vi "Menu Act Language.vi"(8 "error in (no error)":errorcluster, 10 "Language Name":string, 11 "LF2R IDE in":refnum<class "LF2R IDE.lvclass">) -> (0 "error out":errorcluster, 3 "LF2R IDE out":refnum<class "LF2R IDE.lvclass">)   [LabVIEW 2018, in "LF2R IDE.lvlib" / "LF2R IDE.lvclass"]
uses:
  LF2R IDE.lvclass
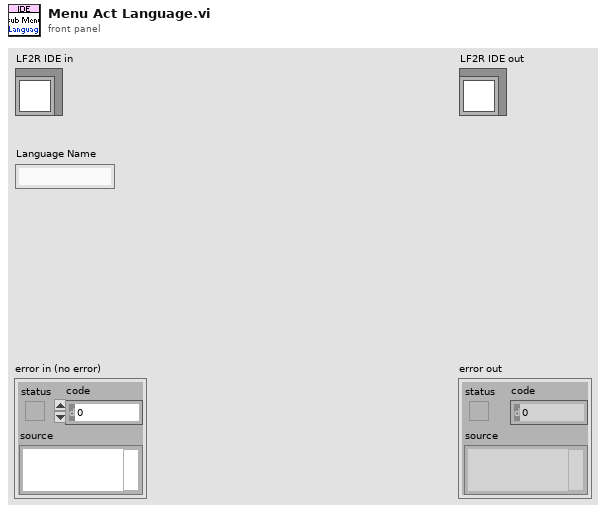
[diagram p1: front panel]
types:
  T1 = typedef "LF2R IDE.lvlib/LF2R IDE.lvclass/Const UI Description Setting.ctl" = cluster{"Title":T2, "Frame Basic":T4, "Frame Skill":T5, "bp":T6, "w":T7, "b":T8, "i":T9, "o":T10, "c":T11, "Other":T12}
  T2 = typedef "LF2R IDE.lvlib/LF2R IDE.lvclass/Const UI Desc Frame Title.ctl" = cluster{"Frame Num":T3, "Name":T3}
  T3 = typedef "LF2R IDE.lvlib/LF2R IDE.lvclass/Const UI Desc Property.ctl" = cluster{"Name":string, "Tip":string}
  T4 = typedef "LF2R IDE.lvlib/LF2R IDE.lvclass/Const UI Desc Frame Basic.ctl" = cluster{"pic":T3, "state":T3, "wait":T3, "next":T3, "dvx":T3, "dvy":T3, "dvz":T3, "centerx":T3, "centery":T3, "sound":T3}
  T5 = typedef "LF2R IDE.lvlib/LF2R IDE.lvclass/Const UI Desc Frame Skill.ctl" = cluster{"mp":T3, "hit_a":T3, "hit_d":T3, "hit_j":T3, "hit_Fa":T3, "hit_Ua":T3, "hit_Da":T3, "hit_Fj":T3, "hit_Uj":T3, "hit_Dj":T3, "hit_ja":T3}
  T6 = typedef "LF2R IDE.lvlib/LF2R IDE.lvclass/Const UI Desc Frame bp.ctl" = cluster{"x":T3, "y":T3}
  T7 = typedef "LF2R IDE.lvlib/LF2R IDE.lvclass/Const UI Desc Frame w.ctl" = cluster{"kind":T3, "x":T3, "y":T3, "weaponact":T3, "cover":T3, "dvx":T3, "dvy":T3, "dvz":T3, "attacking":T3}
  T8 = typedef "LF2R IDE.lvlib/LF2R IDE.lvclass/Const UI Desc Frame b.ctl" = cluster{"kind":T3, "x":T3, "y":T3, "w":T3, "h":T3, "index":T3}
  T9 = typedef "LF2R IDE.lvlib/LF2R IDE.lvclass/Const UI Desc Frame i.ctl" = cluster{"kind":T3, "x":T3, "y":T3, "w":T3, "h":T3, "zwidth":T3, "dvx":T3, "dvy":T3, "dvz":T3, "fall":T3, "arest":T3, "vrest":T3, "bdefend":T3, "injury":T3, "effect":T3, "catchingact 1":T3, "catchingact 2":T3, "caughtact 1":T3, "caughtact 2":T3, "index":T3}
  T10 = typedef "LF2R IDE.lvlib/LF2R IDE.lvclass/Const UI Desc Frame o.ctl" = cluster{"kind":T3, "x":T3, "y":T3, "action":T3, "dvx":T3, "dvy":T3, "dvz":T3, "oid":T3, "facing":T3}
  T11 = typedef "LF2R IDE.lvlib/LF2R IDE.lvclass/Const UI Desc Frame c.ctl" = cluster{"kind":T3, "x":T3, "y":T3, "injury":T3, "cover":T3, "vaction":T3, "aaction":T3, "taction":T3, "hurtable":T3, "decrease":T3, "fronthurtact":T3, "backhurtact":T3, "throwvx":T3, "throwvy":T3, "throwvz":T3, "throwinjury":T3, "dircontrol":T3}
  T12 = typedef "LF2R IDE.lvlib/LF2R IDE.lvclass/Const UI Desc Other.ctl" = cluster{"File Path":T3, "GoTo":T3, "Apply Change":T3, "To Next Frame":T3}
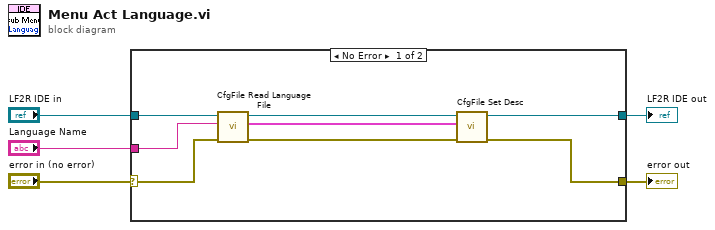
[diagram p0: block diagram]
diagram:
  n1 = case shown="No Error" "error in (no error)" {
    selector: "error in (no error)" -> [w11 w15]
    tunnel: [w6 w15] -> w4
    tunnel: [w7 w14] -> w2
    tunnel: "LF2R IDE in" -> [w13 w14]
    tunnel: "Language Name" -> [w12 _]
    frame No Error {
      n2 = call "CfgFile Read Language File.vi"("error in (no error)"=w11, "Language Name"=w12, "LF2R IDE in"=w13) -> ("error out"=w9:errorcluster, "UI Descriptions"=w8:T1, "LF2R IDE out"=w10:refnum<class "LF2R IDE.lvclass">)  [unwired: 5 in, 1 out]
      n3 = call "CfgFile Set Desc.vi"("error in (no error)"=w9, "UI Descriptions"=w8, "LF2R IDE in"=w10) -> ("error out"=w6:errorcluster, "LF2R IDE out"=w7:refnum<class "LF2R IDE.lvclass">)  [unwired: 7 in]
    }
    frame Error {
    }
  }
  "error out" <- w4
  "LF2R IDE out" <- w2
